vi "FTW-Router-Callback.vi"(4 "Message Queue":T3 {"Routing Rules"."DropTimeout" format="%dmsec"}, 5 "Incoming Message Header":T1 {"RouterID" format="0x%016x"; "Header Pointer" format="0x%016x"; "Message Pointer" format="0x%016x"}, 6 "Incoming Message Event":refnum<user-event>, 7 "Common Event Data":T2) -> ()   [LabVIEW 2014, in "FTW-Router.lvclass"]
uses:
  FTW-Router.lvclass
  FTW-Router-IncomingMessageHeader.ctl
  FTW-Router-CallbackParameters.ctl
  message/FTW-Message.lvclass
  FTW-Router-RoutingRule.ctl
panel:
  out "NULL messages":i32
  out "Messages Handled":i32
  # "Inputs"
  # "Outputs"
  # "Outputs"
  # "This async callback\nhas no outputs"
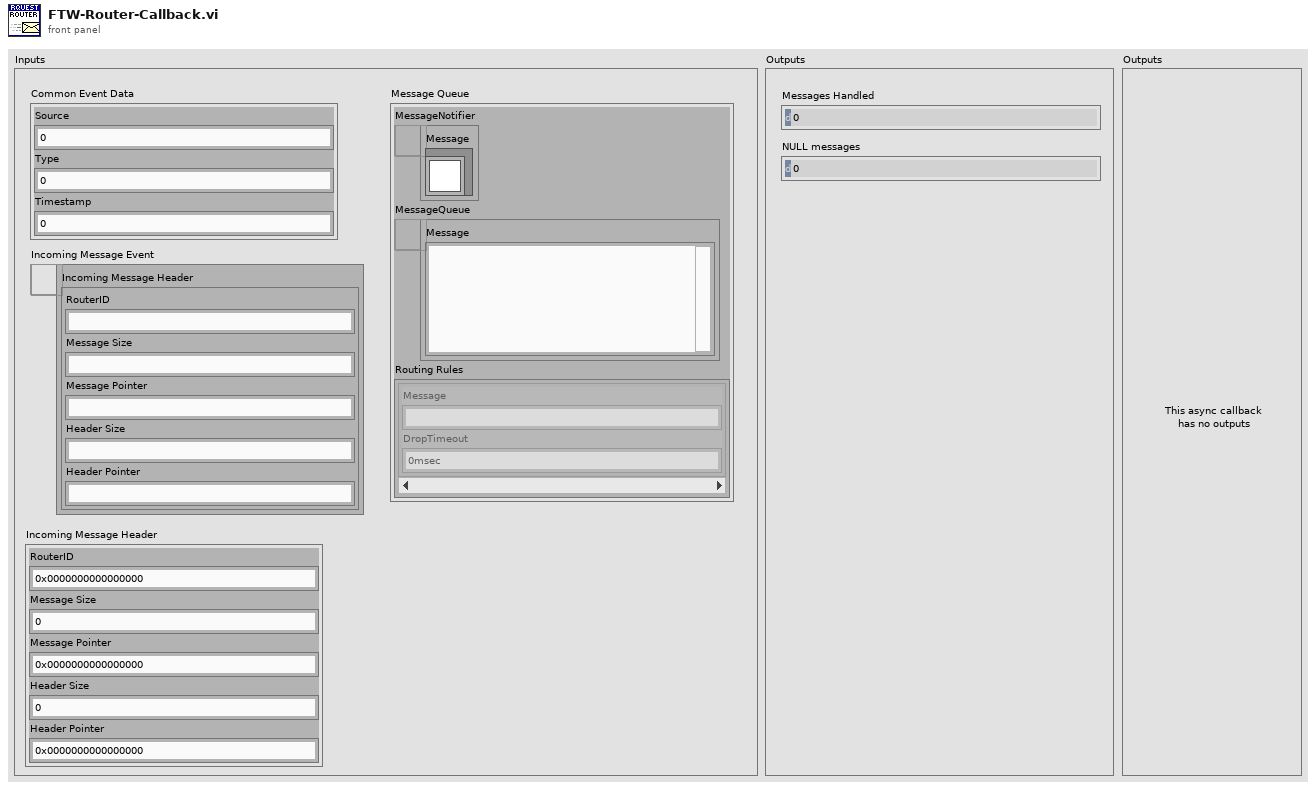
[diagram p1: front panel]
types:
  T1 = typedef "FTW-Router.lvclass/FTW-Router-IncomingMessageHeader.ctl" = cluster{"RouterID":i64, "Message Size":i64, "Message Pointer":i64, "Header Size":i64, "Header Pointer":i64}
  T2 = cluster{"Source":u32, "Type":u32, "Timestamp":u32}
  T3 = typedef "FTW-Router.lvclass/FTW-Router-CallbackParameters.ctl" = cluster{"MessageNotifier":refnum<user-event>, "MessageQueue":refnum<queue>, "Routing Rules":T4[]}
  T4 = typedef "FTW-Router.lvclass/FTW-Router-RoutingRule.ctl" = cluster{"Message":string, "DropTimeout":i32}
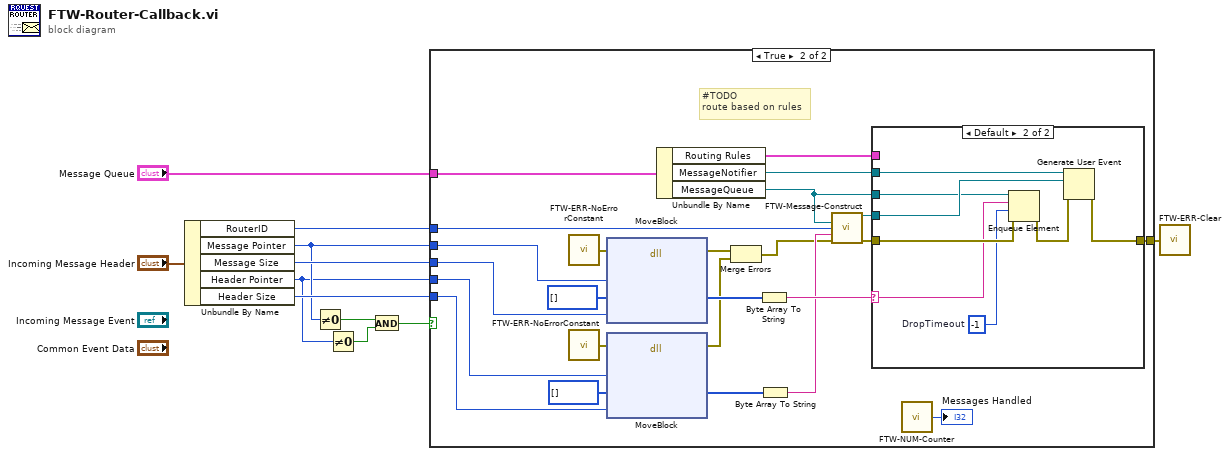
[diagram p0: block diagram]
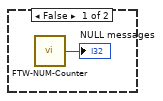
[diagram p2: hidden frame]
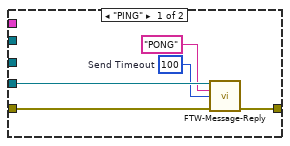
[diagram p3: hidden frame]
diagram:
  n1 = Unbundle By Name("Incoming Message Header") -> ("RouterID"=w6:i64, "Message Pointer"=w5:i64, "Message Size"=w10:i64, "Header Pointer"=w4:i64, "Header Size"=w9:i64)
  n2 = Not Equal To 0?(x=w5) -> (x != 0?=w2:bool)
  n3 = Not Equal To 0?(x=w4) -> (x != 0?=w1:bool)
  n4 = And(x=w2, y=w1) -> (x .and. y?=w3:bool)
  n5 = case shown="True" w3 {
    tunnel: [_ w36] -> w11
    tunnel: w5 -> [_ w33]
    tunnel: w10 -> [_ w32]
    tunnel: w4 -> [_ w29]
    tunnel: w9 -> [_ w28]
    tunnel: "Message Queue" -> [_ w21]
    tunnel: w6 -> [_ w19]
    frame False {
      n6 = call "FTW-NUM-Counter.vi"() -> ("Counter"=→"NULL messages":i32)  [unwired: 1 in]
    }
    frame True {
      # "#TODO\nroute based on rules"
      n7 = call "FTW-ERR-NoErrorConstant.vi"() -> ("no error"=w24:errorcluster)
      n8 = call "FTW-ERR-NoErrorConstant.vi"() -> ("no error"=w25:errorcluster)
      n9 = dll-call lib="LabVIEW" fn="MoveBlock"(error in=w24, "Source Pointer"=w33, "Destination"=u8[] [], "Length"=w32) -> (error out=w23:errorcluster, "Destination"=w26:u8[])  [unwired: 5 in, 1 out]
      n10 = dll-call lib="LabVIEW" fn="MoveBlock"(error in=w25, "Source Pointer"=w29, "Destination"=u8[] [], "Length"=w28) -> (error out=w22:errorcluster, "Destination"=w27:u8[])  [unwired: 5 in, 1 out]
      n11 = Unbundle By Name(w21) -> ("Routing Rules"=w13:T4[], "MessageNotifier"=w18:refnum<user-event>, "MessageQueue"=w15:refnum<queue>)
      n12 = Merge Errors(w23, w22) -> (w14:errorcluster)
      n13 = Byte Array To String(unsigned byte array=w26) -> (string=w17:string)
      n14 = Byte Array To String(unsigned byte array=w27) -> (string=w16:string)
      n15 = call "FTW-Message-Construct.vi"("MessageQueue"=w15, "SocketID"=w19, "Headers"=w16, "error in"=w14) -> ("FTW Incoming Message"=w35:refnum<class "FTW-Message.lvclass">, "error out"=w34:errorcluster)  [unwired: 10 in]
      n16 = case shown="Default" w17 {
        selector: w17 -> [_ w42]
        tunnel: [w37 w49] -> w36
        tunnel: w35 -> [w41 w48]
        tunnel: w34 -> [w38 w45]
        tunnel: w18 -> [_ w47]
        tunnel: w15 -> [_ w46]
        tunnel: w13 -> [_ _]
        frame "PING" {
          w39 = 100  # Send Timeout
          n17 = call "FTW-Message-Reply.vi"("FTW Incoming Message"=w41, "Response"="PONG", "Send Timeout"=w39, "error in"=w38) -> ("error out"=w37:errorcluster)  [unwired: 10 in, 1 out]
        }
        frame Default {
          w43 = -1  # DropTimeout
          n18 = Enqueue Element(queue=w46, element=w42, timeout in ms (-1)=w43, error in (no error)=w45) -> (error out=w44:errorcluster)  [unwired: 2 out]
          n19 = Generate User Event(user event=w47, event data cluster=w48, error in=w44) -> (error out=w49:errorcluster)  [unwired: 1 in, 1 out]
        }
      }
      n20 = call "FTW-NUM-Counter.vi"() -> ("Counter"=→"Messages Handled":i32)  [unwired: 1 in]
    }
  }
  n21 = call "FTW-ERR-Clear.vi"("error to snuff"=w11) -> ()  [unwired: 1 out]
